vi "Paint Bounding Box[CoolerBot].vi"(9 "Camera Image":T5) -> (0 "Thresholded Image":T5(plugin-control), 1 "Center of Mass":cluster{"X":dbl, "Y":dbl}, 2 "Area":dbl, 3 "Particle Report":T3, 4 "General Report":T4(array[cluster]))   [LabVIEW 2016]
uses:
  <vilib>/vision/Image Controls.llb/IMAQ Image.ctl
panel:
  out "The Chosen One":T1
  out "General Circles":T2(array[cluster])
  out "Circles":T2(array[cluster]) {"Position"."Y" format="%.2f"; "Position"."X" format="%.2f"}
  in  "R/G/B":cluster{"Lower value":i32, "Upper value":i32}[](array[cluster])=[{"Lower value"=0, "Upper value"=40}, {"Lower value"=80, "Upper value"=255}, {"Lower value"=0, "Upper value"=255}]
  out "Particle Report":T4(array[cluster]) {"Orientation" format="%.2f"; "Dimensions"."Height" format="%.2f"; "Dimensions"."Width" format="%.2f"; "Center of Mass"."Y" format="%.2f"; "Center of Mass"."X" format="%.2f"; "Bounding Rect"."Bottom" format="%.2f"; "Bounding Rect"."Right" format="%.2f"; "Bounding Rect"."Top" format="%.2f"; "Bounding Rect"."Left" format="%.2f"; "Number of Holes" format="%.2f"; "Area" format="%.2f"}
  in  "sampleimage":string
  out "Base Image":T5(plugin-control)
  # "difference = width*4"
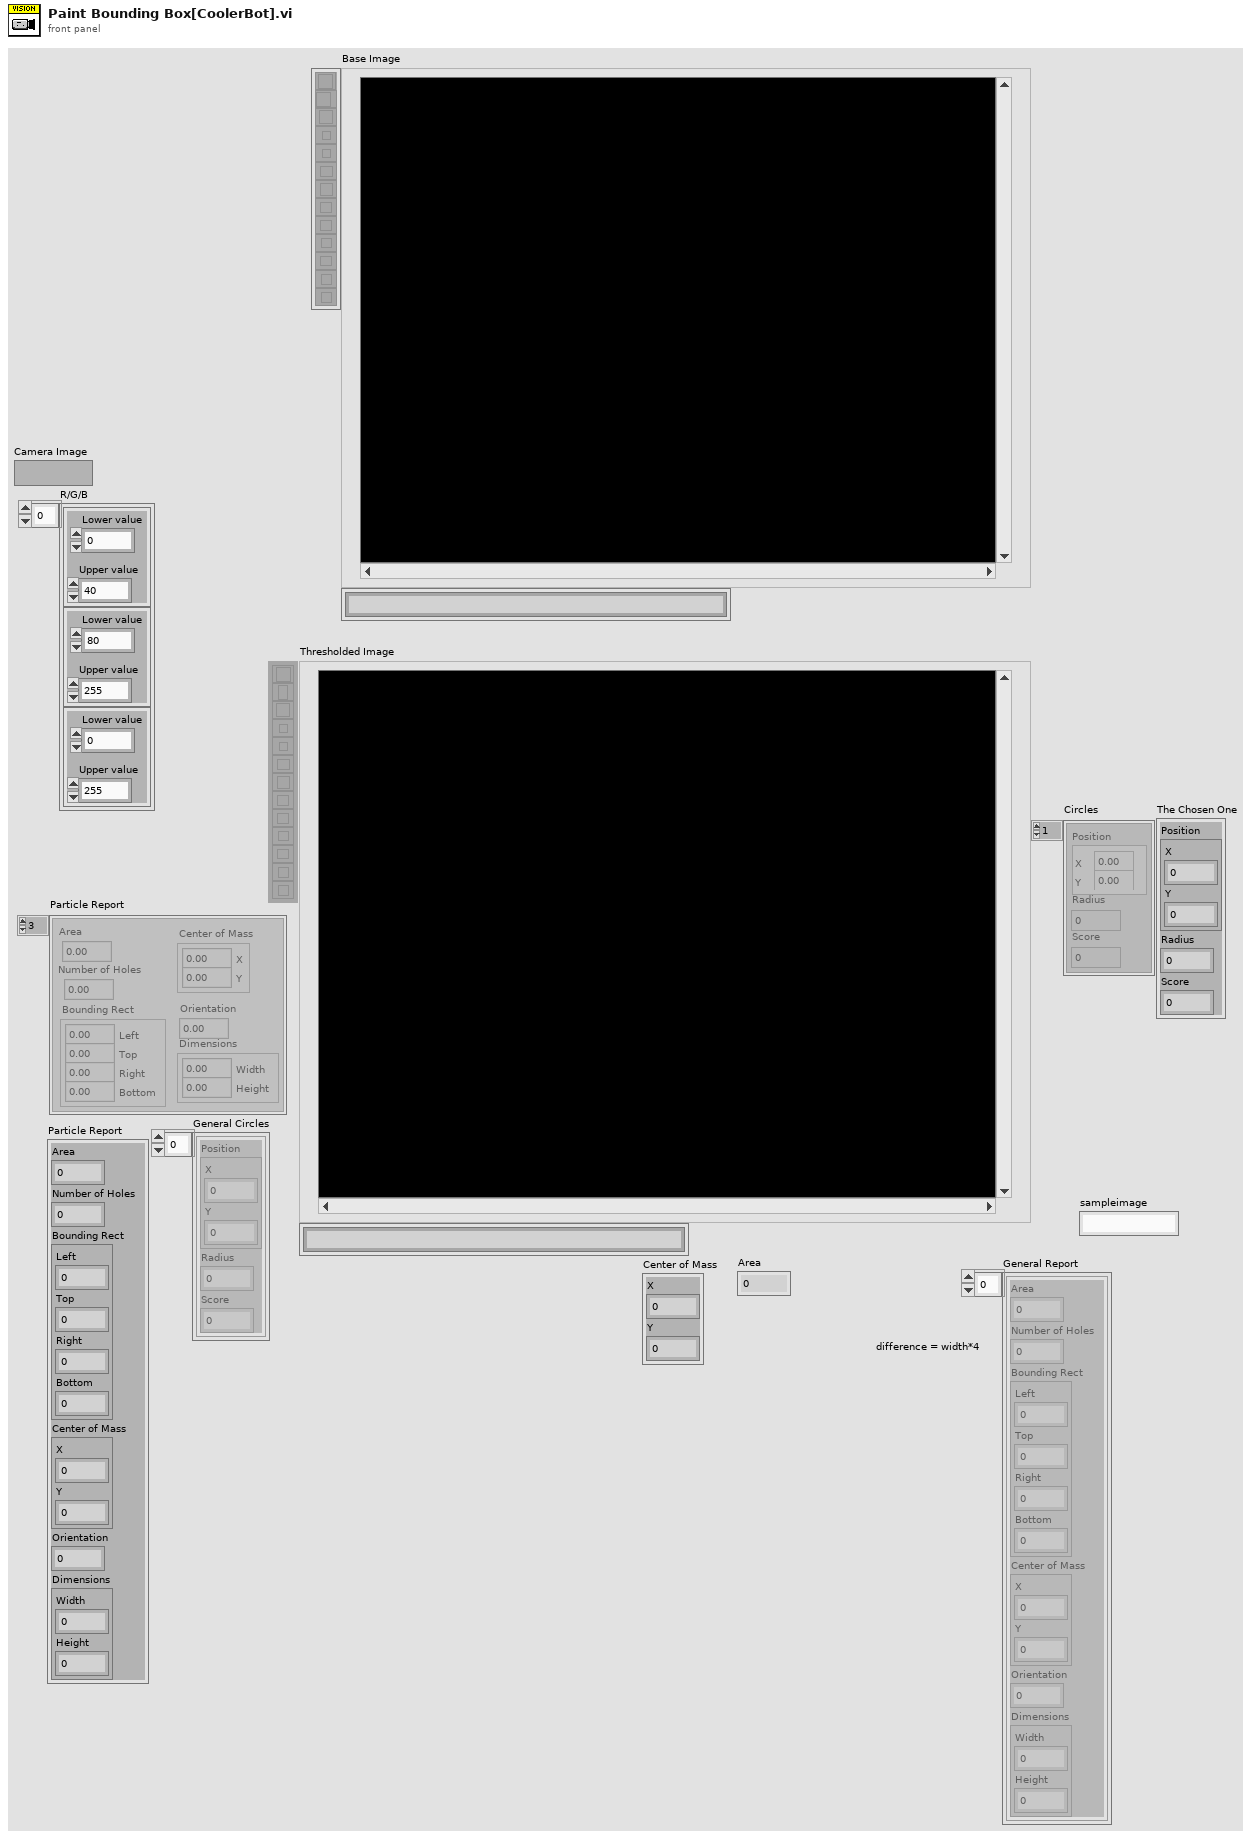
[diagram p1: front panel]
types:
  T1 = cluster{"Position":cluster{"X":sgl, "Y":sgl}, "Radius":dbl, "Score":dbl}
  T2 = cluster{"Position":cluster{"X":sgl, "Y":sgl}, "Radius":dbl, "Score":dbl}[]
  T3 = cluster{"Area":dbl, "Number of Holes":dbl, "Bounding Rect":cluster{"Left":dbl, "Top":dbl, "Right":dbl, "Bottom":dbl}, "Center of Mass":cluster{"X":dbl, "Y":dbl}, "Orientation":dbl, "Dimensions":cluster{"Width":dbl, "Height":dbl}}
  T4 = cluster{"Area":dbl, "Number of Holes":dbl, "Bounding Rect":cluster{"Left":dbl, "Top":dbl, "Right":dbl, "Bottom":dbl}, "Center of Mass":cluster{"X":dbl, "Y":dbl}, "Orientation":dbl, "Dimensions":cluster{"Width":dbl, "Height":dbl}}[]
  T5 = typedef "IMAQ Image.ctl" = refnum<image>
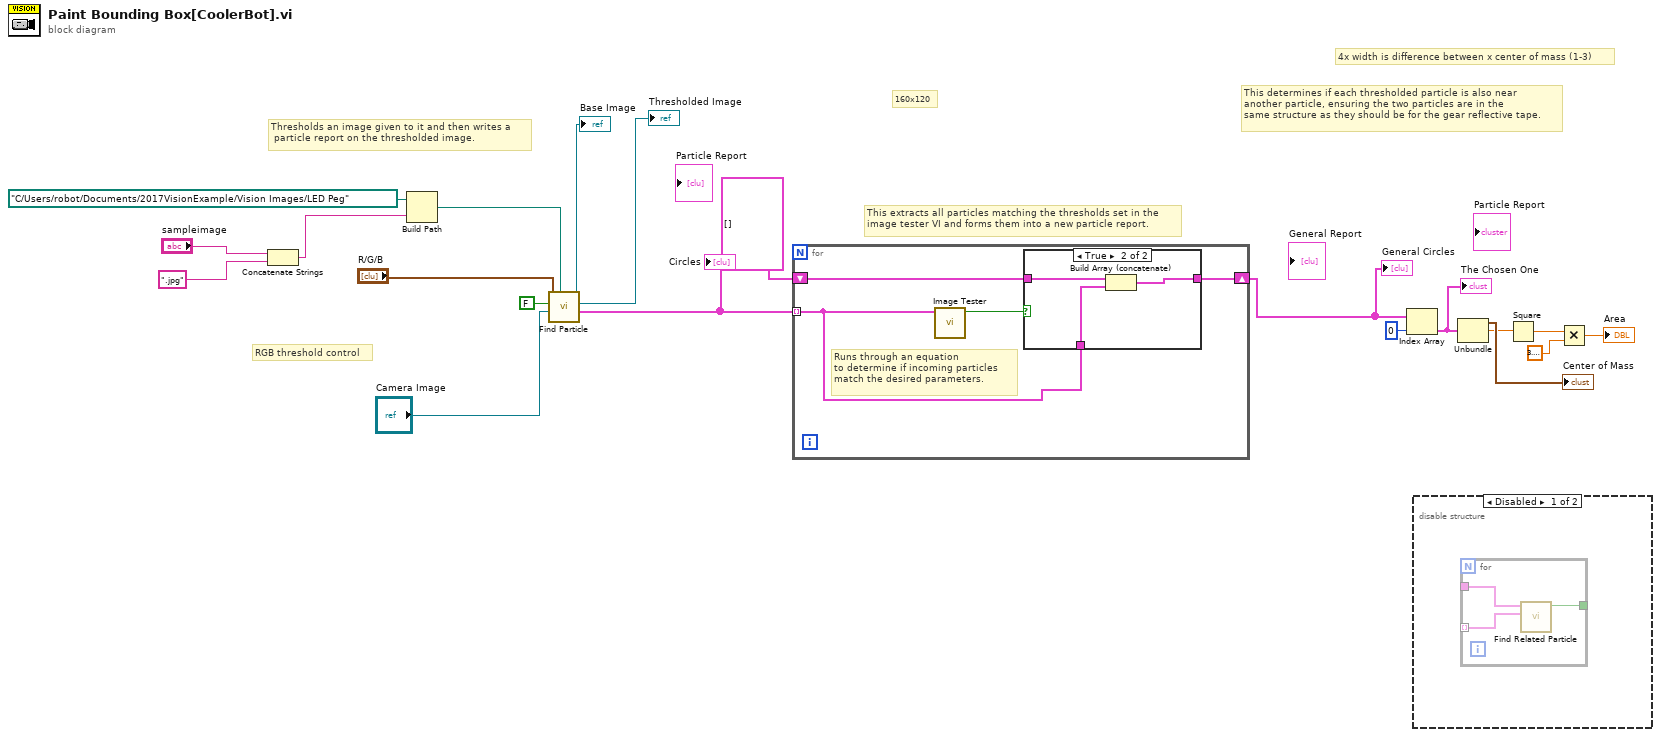
[diagram p0: block diagram]
diagram:
  # "This determines if each thresholded particle is also near \nanother particle, ensuring the two particles are in the \nsame structure as they should be for the gear reflective tape."
  # "4x width is difference between x center of mass (1-3)"
  # "RGB threshold control"
  # "This extracts all particles matching the thresholds set in the \nimage tester VI and forms them into a new particle report."
  # "Thresholds an image given to it and then writes a\n particle report on the thresholded image."
  # "160x120"
  n1 = Concatenate Strings("sampleimage", ".jpg" ("string")) -> (w12:string)
  n2 = Build Path(base path=path "C:/Users/robot/Documents/2017VisionExample/Vision Images/LED Peg", name or relative path=w12) -> (appended path=w13:path)
  n3 = call "Find Particle.vi"("File Path"=w13, "Camera Image"="Camera Image", "From File"=FALSE, "R/G/B"="R/G/B") -> ("Circles"=w19:T2, "Thresholded Image"=→"Thresholded Image":T5, "Base Image"=→"Base Image":T5)  [unwired: 3 in, 2 out]
  "Circles" <- w19
  n4 = for {
    tunnel: w19 -> [w21] mode=indexing
    shift-right: [w24] -> w2
    shift-left: T2 [] ("Circles") -> [w23]
    # "Runs through an equation\nto determine if incoming particles \nmatch the desired parameters."
    n5 = call "Image Tester.vi"("Circle Descriptor"=w21) -> ("Positive"=w22:bool)  [unwired: 10 in]
    n6 = case shown="True" w22 {
      tunnel: w21 -> [_ w26]
      tunnel: [w25 w28] -> w24
      tunnel: w23 -> [w25 w27]
      frame False {
      }
      frame True {
        n7 = Build Array (concatenate)(w27, w26) -> (w28:T2)
      }
    }
  }
  "General Circles" <- w2
  n8 = Index Array(array=w2, index=0) -> (element=w8:T1)
  "The Chosen One" <- w8
  n9 = disable-structure shown="Disabled" {
    frame Disabled {
      n10 = for {
        tunnel: _ -> [w31]
        tunnel: _ -> [w30] mode=indexing
        tunnel: [w29] -> _
        n11 = call "Find Related Particle.vi"("All Reports"=w30, "Base Report"=w31) -> ("Nearby"=w29:bool)  [unwired: 9 in]
      }
    }
    frame Enabled {
    }
  }
  n12 = Unbundle(w8) -> ("Position"=→"Center of Mass":cluster{"X":sgl, "Y":sgl}, "Radius"=w4:dbl)  [unwired: 1 out]
  n13 = Square(x=w4) -> (x^2=w6:dbl)
  n14 = Multiply(x=w6, y=3.141592653589793) -> (x*y=→"Area":dbl)
